vi "EOG_cancel_Method.vi"() -> ()   [LabVIEW 2014]
uses:
  <vilib>/Analysis/3filter.llb/Filter Passband Type.ctl
  <vilib>/Analysis/baseanly.llb/Real A x B.vi
  <vilib>/Utility/file.llb/Read From Spreadsheet File (DBL).vi
  <vilib>/Utility/file.llb/Read From Spreadsheet File (I64).vi
  <vilib>/Analysis/3filter.llb/Butterworth Filter (DBL).vi
  <vilib>/Analysis/Matrix/Numeric/Absolute Value/Absolute Value - RM.vi
  <vilib>/Analysis/Matrix/Numeric/Conversions/Matrix To Array - RM.vi
  <vilib>/Analysis/NI_AALBase.lvlib
  <vilib>/gmath/NI_Gmath.lvlib
  <vilib>/Analysis/Matrix/NI_Matrix.lvlib
panel:
  out "Revised 2":dbl[][](graph)
  in  "Cluster":path
  out "Revised":dbl[](graph)
  in  "Inverse_W":path
  out "Trans\nSTFT":dbl[][](graph)
  out "STFT":dbl[][](graph)
  in  "Exit":bool
  in  "Continuous/Discreet":bool
  in  "Forward":bool
  in  "Pause":bool
  out "STD Method":bool
  out "Cancel out \n(Std method)":dbl[](graph)
  out "Original":bool
  out "EEG":dbl[](graph)
  in  "Process":bool
  out "Processing":bool
  in  "Trial Number":i32=1
  in  "?":bool
  in  "Frame_Length":i32=20
  in  "Flash_Repeat":i32=20
  in  "Random_num":i32=6
  in  "EEG Data":path
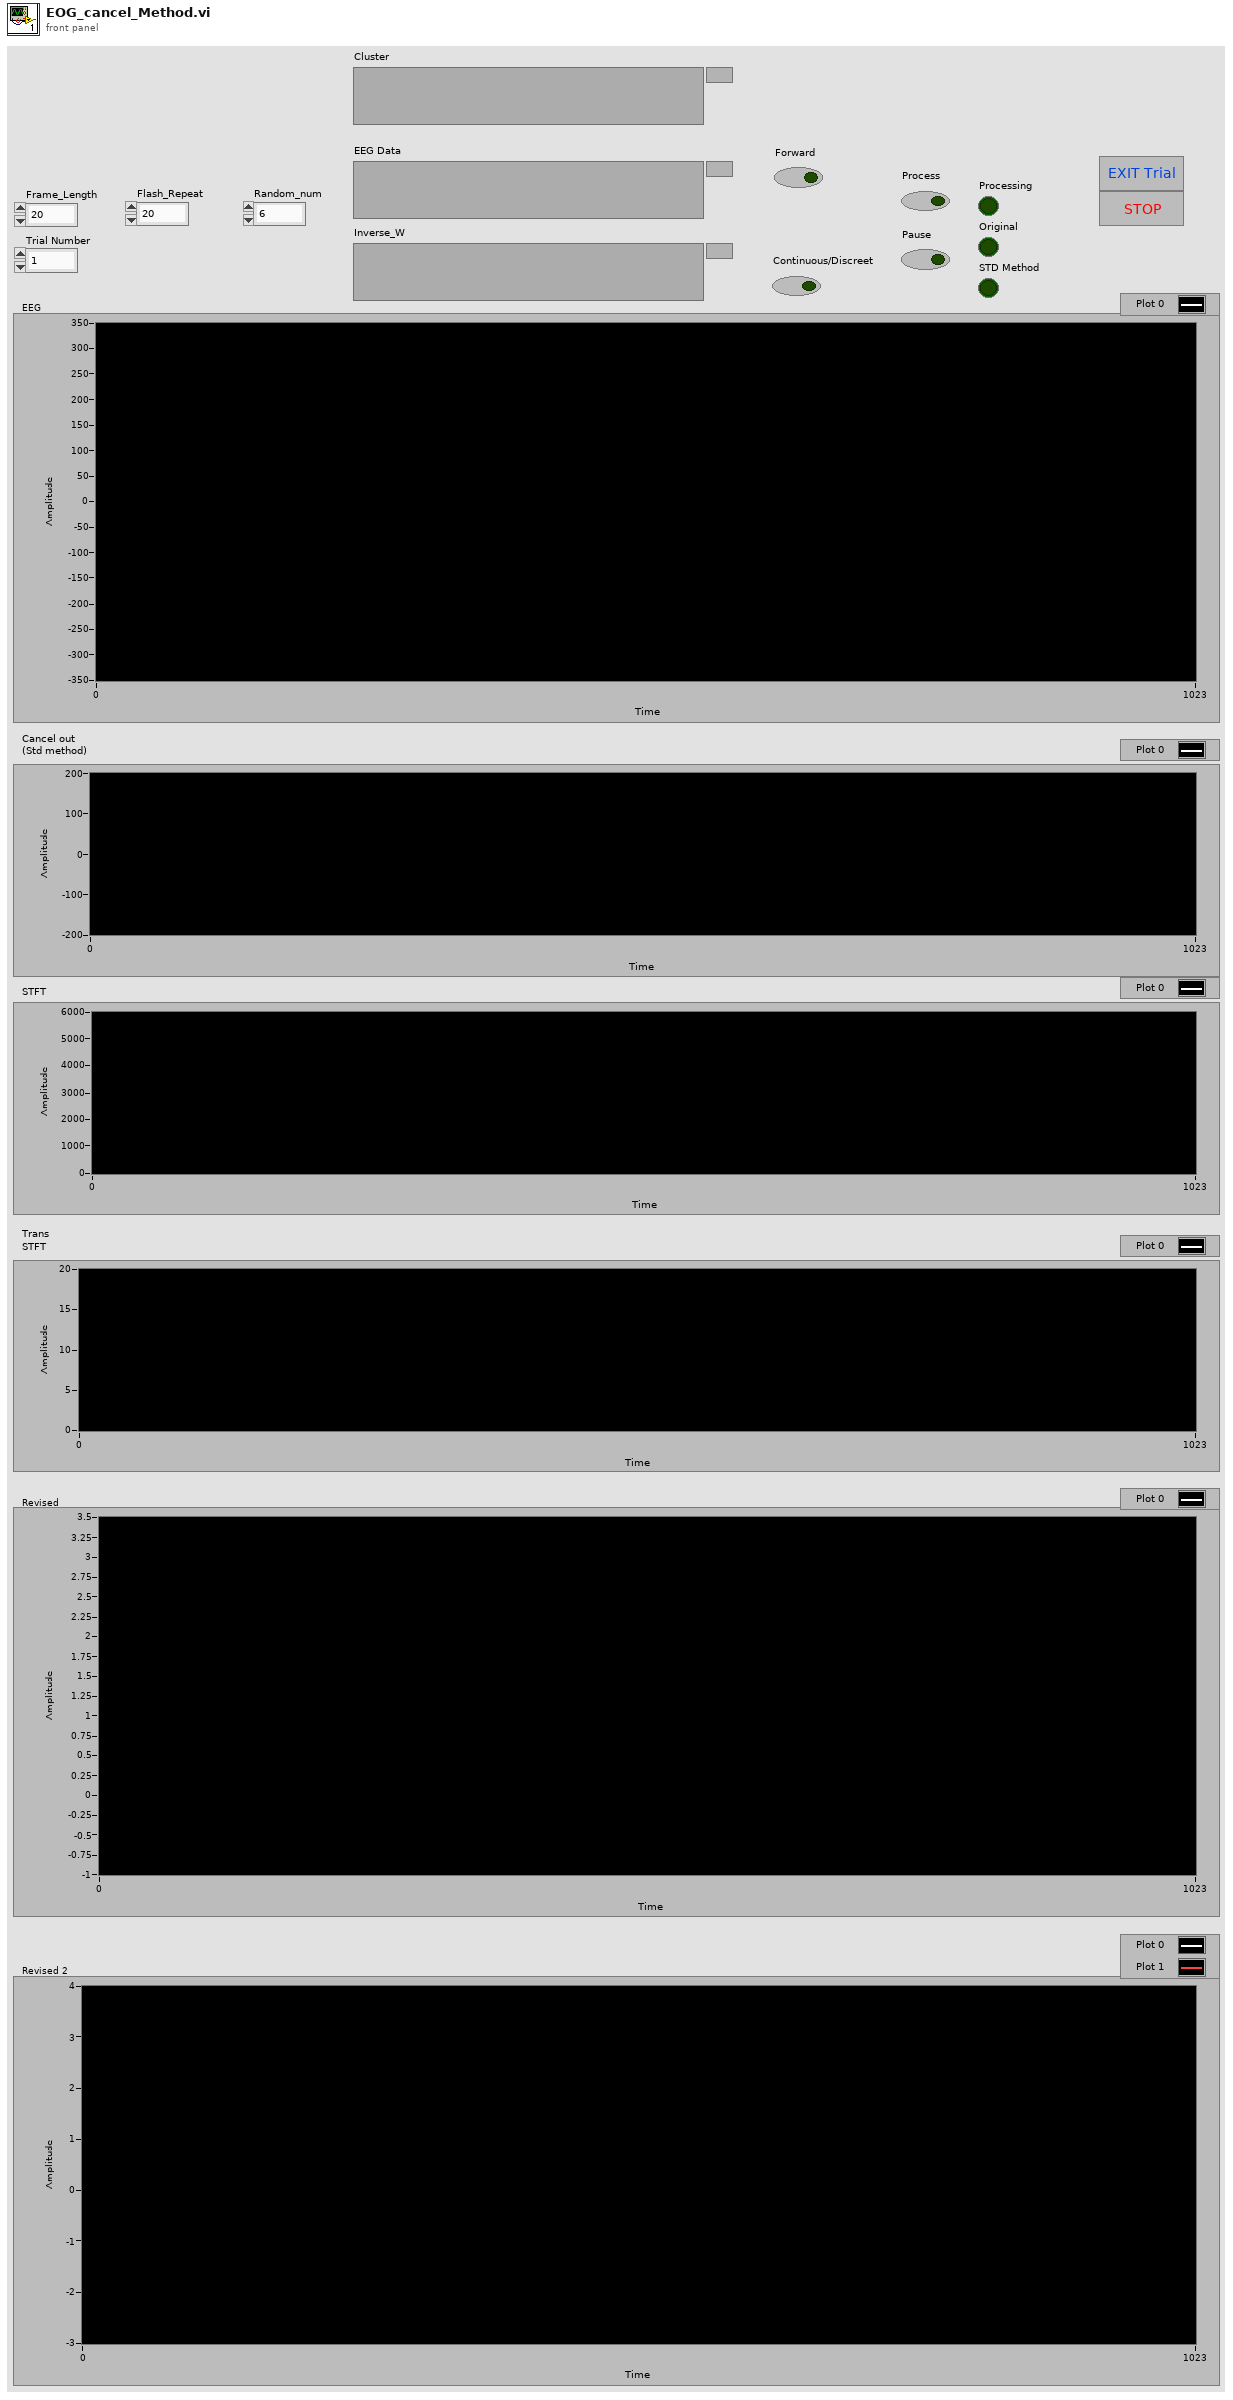
[diagram p1: front panel]
types:
  T1 = typedef "NI_AALBase.lvlib/Filter Passband Type.ctl" = enum32{"Lowpass", "Highpass", "Bandpass", "Bandstop"}
  T2 = typedef "NI_Matrix.lvlib/RealMatrix.ctl" = dbl[][]
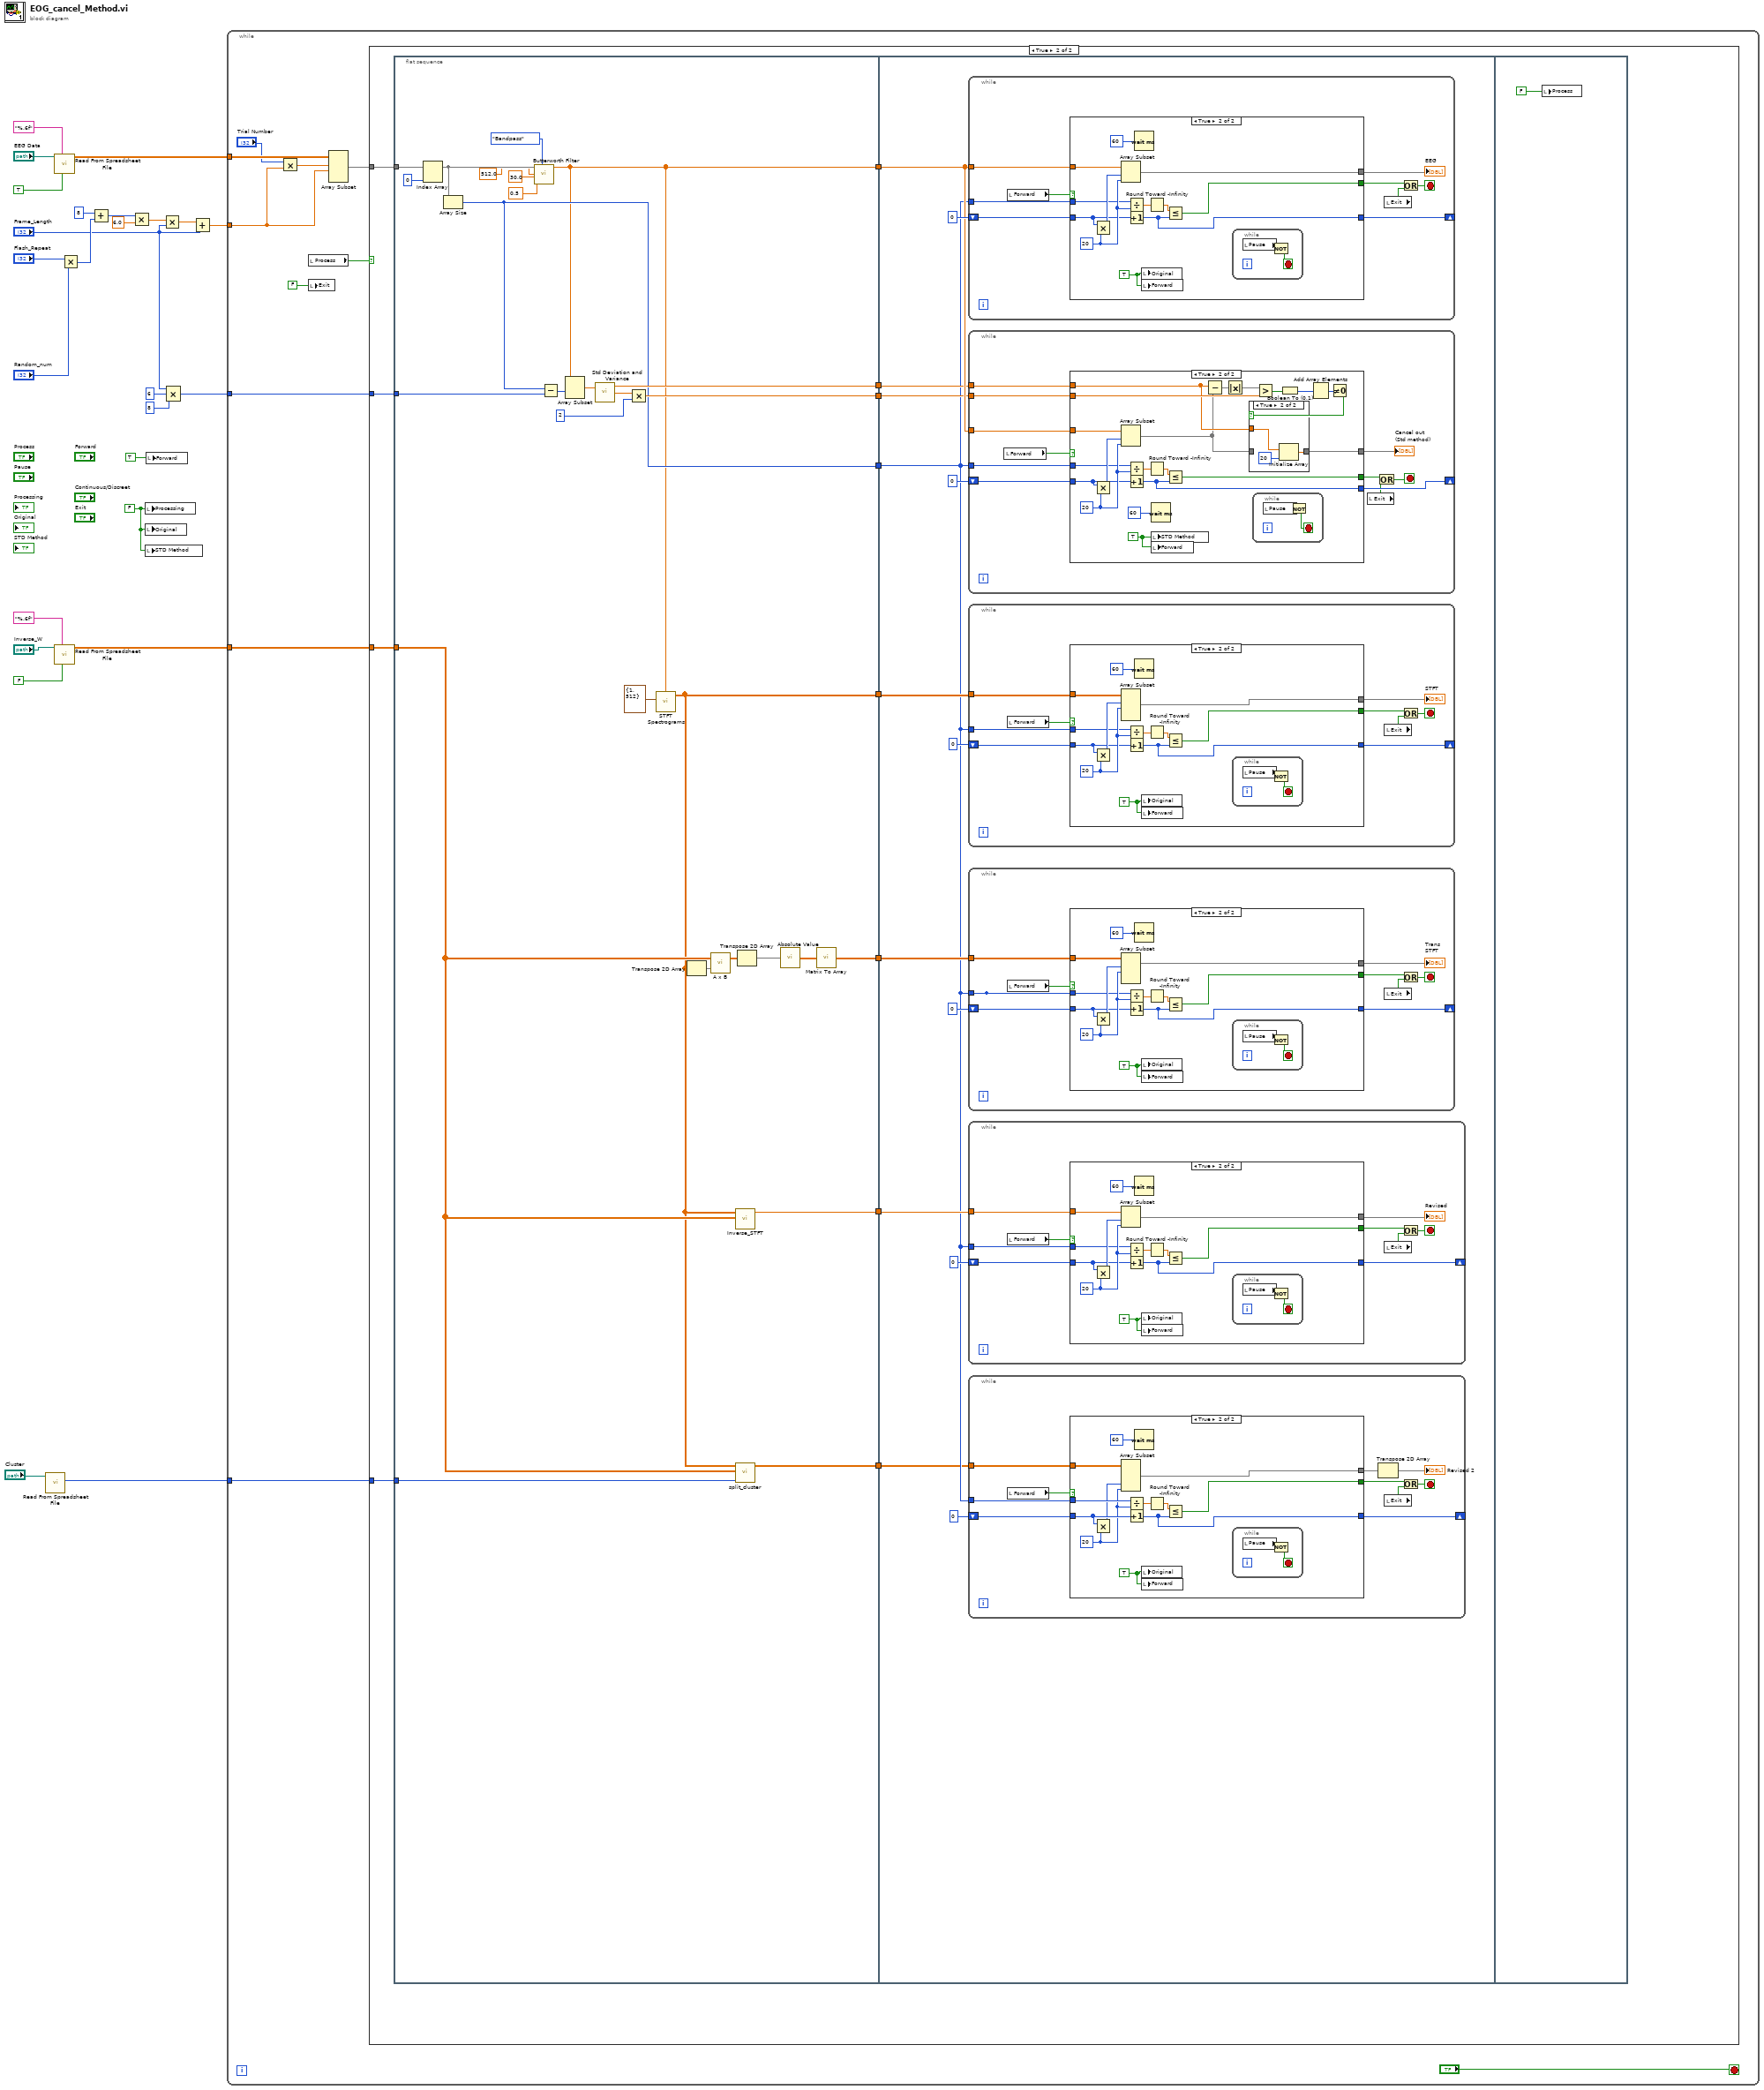
[diagram p0: block diagram]
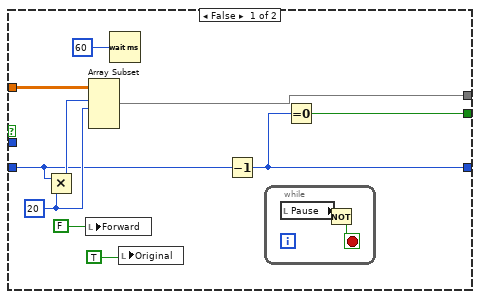
[diagram p3: hidden frame]
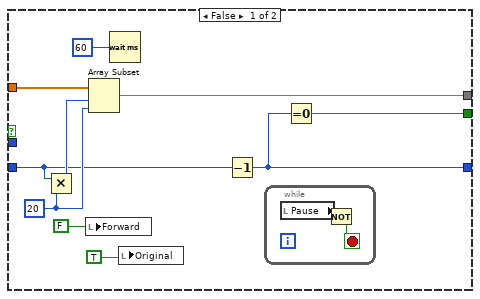
[diagram p4: hidden frame]
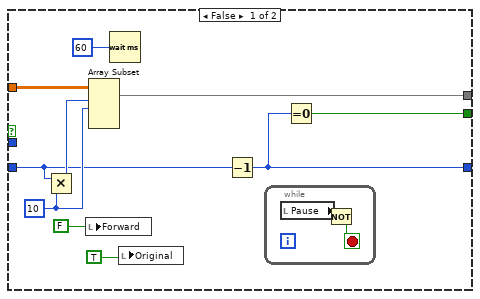
[diagram p5: hidden frame]
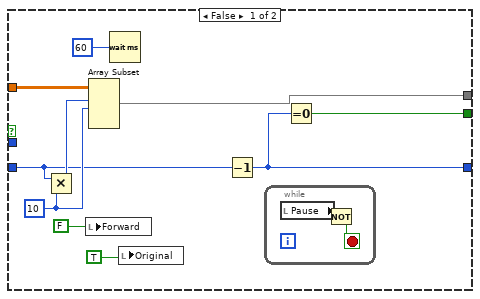
[diagram p6: hidden frame]
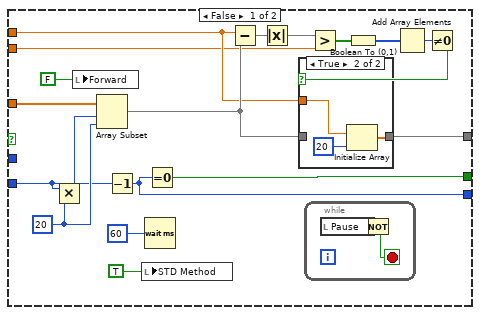
[diagram p7: hidden frame]
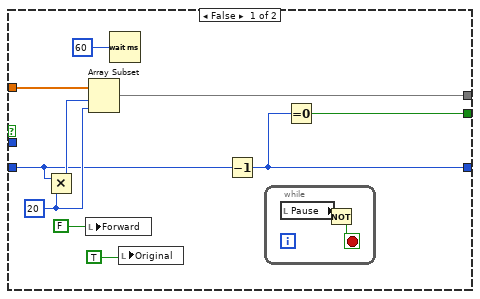
[diagram p10: hidden frame]
diagram:
  w7 = FALSE ("Processing")
  n1 = call-poly <vilib>:"Read From Spreadsheet File.vi"("file path (dialog if empty)"="Cluster") -> ("first row"=w1:i64[])  [unwired: 6 in, 4 out]
  n2 = call-poly <vilib>:"Read From Spreadsheet File.vi"("transpose (no:F)"=TRUE, "format (%.3f)"="%.6f", "file path (dialog if empty)"="EEG Data") -> ("all rows"=w13:dbl[][])  [unwired: 4 in, 4 out]
  n3 = call-poly <vilib>:"Read From Spreadsheet File.vi"("transpose (no:F)"=FALSE, "format (%.3f)"="%.6f", "file path (dialog if empty)"="Inverse_W") -> ("all rows"=w3:dbl[][])  [unwired: 4 in, 4 out]
  n4 = Multiply(x="Flash_Repeat", y="Random_num") -> (x*y=w17:i32)
  n5 = Add(x=8, y=w17) -> (x+y=w19:i32)
  n6 = Multiply(x=w19, y=6.0) -> (x*y=w21:dbl)
  n7 = local write "Processing"(w7) -> ()
  n8 = local write "Original"(w7) -> ()
  n9 = local write "STD Method"(w7) -> ()
  n10 = local write "Forward"(TRUE ("Forward")) -> ()
  n11 = Multiply(x=w21, y="Frame_Length") -> (x*y=w22:dbl)
  n12 = Compound Arithmetic op=MULTIPLY("Frame_Length", 6 ("x"), 8 ("x")) -> (w9:i32)
  n13 = Add(x=w22, y="Frame_Length") -> (x+y=w14:dbl)
  n14 = while {
    tunnel: w13 -> [w35]
    tunnel: w14 -> [w33]
    tunnel: w9 -> [w30]
    tunnel: w3 -> [w27]
    tunnel: w1 -> [w26]
    stop <- "?" stop-if-true
    n15 = Multiply(x="Trial Number", y=w33) -> (x*y=w34:dbl)
    n16 = local read "Process"() -> (w29:bool)
    n17 = local write "Exit"(FALSE ("Exit")) -> ()
    n18 = Array Subset(array=w35, index (row)=w34, length (row)=w33) -> (w31:dbl[][])  [unwired: 2 in]
    n19 = case shown="True" w29 {
      tunnel: w31 -> [_ w47]
      tunnel: w30 -> [_ w48]
      tunnel: w27 -> [_ w46]
      tunnel: w26 -> [_ w38]
      frame False {
      }
      frame True {
        n20 = flat-sequence {
          tunnel: w48 -> [w75]
          tunnel: w47 -> [w74]
          tunnel: w46 -> [w50]
          tunnel: [w70] -> w45
          tunnel: [w69] -> w44
          tunnel: [w61] -> w43
          tunnel: [w59] -> w42
          tunnel: [w49] -> w41
          tunnel: [w53] -> w40
          tunnel: [w55] -> w39
          tunnel: w38 -> [w52]
          tunnel: [w51] -> w37
          tunnel: w45 -> [w84]
          tunnel: w44 -> [w85]
          tunnel: w43 -> [w77]
          tunnel: w42 -> [w86]
          tunnel: w41 -> [w83]
          tunnel: w40 -> [w82]
          tunnel: w39 -> [w79]
          tunnel: w37 -> [w76]
          frame #0 {
            n21 = Index Array(array=w74, index (col)=0 ("disabled index (col)")) -> (element=w64:dbl[])  [unwired: 1 in]
            n22 = Array Size(array=w64) -> (size(s)=w61:i32)
            n23 = call-poly <vilib>:"Butterworth Filter.vi"("filter type"=Filter_Passband_Type."Bandpass", "low cutoff freq: fl"=0.5, "high cutoff freq: fh"=30.0, "sampling freq: fs"=512.0 ("high cutoff freq: fh"), "X"=w64) -> ("Filtered X"=w59:dbl[])  [unwired: 3 in, 1 out]
            n24 = Subtract(x=w61, y=w75) -> (x-y=w73:i32)
            n25 = Array Subset(array=w59, index=w73) -> (w62:dbl[])  [unwired: 1 in]
            n26 = call <vilib>:"Std Deviation and Variance.vi"("X"=w62) -> ("mean"=w69:dbl, "standard deviation"=w72:dbl)  [unwired: 1 in, 1 out]
            n27 = Multiply(x=w72, y=2 ("disabled index (col)")) -> (x*y=w70:dbl)
            n28 = call <vilib>:"STFT Spectrograms.vi"("time-freq sampling info"=cluster{"time steps":i32, "frequency bins":i32} {"time steps"=1, "frequency bins"=512}, "X"=w59) -> ("STFT Spectrogram {X}"=w49:dbl[][])  [unwired: 8 in, 1 out]
            n29 = Transpose 2D Array(2D array=w49) -> (transposed array=w58:dbl[][])
            n30 = call-poly <vilib>:"A x B.vi"("B"=w58, "A"=w50) -> ("A x B"=w56:T2)  [unwired: 1 out]
            n31 = call "Inverse_STFT.vi"("W"=w50, "STFT Spectrogram {X}"=w49) -> ("Inverse_STFT"=w55:dbl[])  [unwired: 9 in]
            n32 = call "split_cluster.vi"("Clustering"=w52, "W"=w50, "STFT Spectrogram {X}"=w49) -> ("Splited_X(t)"=w51:dbl[][])  [unwired: 7 in, 1 out]
            n33 = Transpose 2D Array(2D array=w56) -> (transposed array=w57:T2)
            n34 = call-poly <vilib>:"Absolute Value.vi"("Real Matrix A"=w57) -> ("|A|"=w54:T2)
            n35 = call-poly <vilib>:"Matrix To Array.vi"("Real Matrix"=w54) -> ("Real 2D Array"=w53:dbl[][])
          }
          frame #1 {
            n36 = while {
              tunnel: w86 -> [w302]
              tunnel: w77 -> [w301]
              shift-right: [w299] -> _
              shift-left: 0 ("disabled index (col)") -> [w300]
              stop <- w297 stop-if-true
              n37 = local read "Forward"() -> (w294:bool)
              n38 = case shown="True" w294 {
                tunnel: w302 -> [w309 w326]
                tunnel: w301 -> [_ w321]
                tunnel: [w306 w320] -> w296
                tunnel: w300 -> [w307 w318]
                tunnel: [w305 w316] -> w299
                tunnel: [w308 w317] -> w298
                frame False {
                  w311 = 20
                  n39 = Multiply(x=w307, y=w311) -> (x*y=w312:i32)
                  n40 = local write "Forward"(FALSE ("Forward")) -> ()
                  n41 = Array Subset(array=w309, index=w312, length=w311) -> (w308:dbl[])
                  n42 = Wait (ms)(milliseconds to wait=u32 60) -> ()  [unwired: 1 out]
                  n43 = local write "Original"(TRUE ("Processing")) -> ()
                  n44 = Decrement(x=w307) -> (x-1=w305:i32)
                  n45 = while {
                    stop <- w313 stop-if-true
                    n46 = local read "Pause"() -> (w314:bool)
                    n47 = Not(x=w314) -> (.not. x?=w313:bool)
                  }
                  n48 = Equal To 0?(x=w305) -> (x = 0?=w306:bool)
                }
                frame True {
                  w315 = TRUE ("Processing")
                  w322 = 20
                  n49 = Multiply(x=w318, y=w322) -> (x*y=w325:i32)
                  n50 = Array Subset(array=w326, index=w325, length=w322) -> (w317:dbl[])
                  n51 = Divide(x=w321, y=w322) -> (x/y=w323:dbl)
                  n52 = Increment(x=w318) -> (x+1=w316:i32)
                  n53 = Wait (ms)(milliseconds to wait=u32 60) -> ()  [unwired: 1 out]
                  n54 = local write "Original"(w315) -> ()
                  n55 = local write "Forward"(w315) -> ()
                  n56 = Round Toward -Infinity(1:w323) -> (0:w324:dbl)
                  n57 = Less Or Equal?(x=w324, y=w316) -> (x <= y?=w320:bool)
                  n58 = while {
                    stop <- w327 stop-if-true
                    n59 = local read "Pause"() -> (w328:bool)
                    n60 = Not(x=w328) -> (.not. x?=w327:bool)
                  }
                }
              }
              "EEG" <- w298
              n61 = local read "Exit"() -> (w295:bool)
              n62 = Or(x=w296, y=w295) -> (x .or. y?=w297:bool)
            }
            n63 = while {
              tunnel: w86 -> [w241]
              tunnel: w77 -> [w240]
              tunnel: w84 -> [w238]
              tunnel: w85 -> [w237]
              shift-right: [w235] -> _
              shift-left: 0 ("disabled index (col)") -> [w236]
              stop <- w233 stop-if-true
              n64 = local read "Forward"() -> (w231:bool)
              n65 = case shown="True" w231 {
                tunnel: w241 -> [w248 w287]
                tunnel: w240 -> [_ w282]
                tunnel: [w244 w281] -> w234
                tunnel: [w247 w279] -> w239
                tunnel: w238 -> [w250 w276]
                tunnel: w237 -> [w251 w271]
                tunnel: w236 -> [w246 w269]
                tunnel: [w245 w268] -> w235
                frame False {
                  w259 = 20
                  n66 = Multiply(x=w246, y=w259) -> (x*y=w260:i32)
                  n67 = local write "Forward"(FALSE ("Forward")) -> ()
                  n68 = Array Subset(array=w248, index=w260, length=w259) -> (w252:dbl[])
                  n69 = Decrement(x=w246) -> (x-1=w245:i32)
                  n70 = local write "STD Method"(TRUE ("Processing")) -> ()
                  n71 = Wait (ms)(milliseconds to wait=u32 60) -> ()  [unwired: 1 out]
                  n72 = Equal To 0?(x=w245) -> (x = 0?=w244:bool)
                  n73 = Subtract(x=w252, y=w251) -> (x-y=w257:dbl[])
                  n74 = Absolute Value(x=w257) -> (abs(x)=w256:dbl[])
                  n75 = while {
                    stop <- w261 stop-if-true
                    n76 = local read "Pause"() -> (w262:bool)
                    n77 = Not(x=w262) -> (.not. x?=w261:bool)
                  }
                  n78 = Greater?(x=w256, y=w250) -> (0:w255:bool[])
                  n79 = Boolean To (0,1)(Boolean=w255) -> (0, 1=w249:i16[])
                  n80 = Add Array Elements(numeric array=w249) -> (sum=w254:i16)
                  n81 = Not Equal To 0?(x=w254) -> (x != 0?=w253:bool)
                  n82 = case shown="True" w253 {
                    tunnel: w252 -> [w263 _]
                    tunnel: [w263 w266] -> w247
                    tunnel: w251 -> [_ w264]
                    frame False {
                    }
                    frame True {
                      n83 = Initialize Array(w264, 20 ("dimension size")) -> (w266:dbl[])
                    }
                  }
                }
                frame True {
                  w267 = TRUE ("Processing")
                  w283 = 20
                  n84 = Multiply(x=w269, y=w283) -> (x*y=w286:i32)
                  n85 = Array Subset(array=w287, index=w286, length=w283) -> (w270:dbl[])
                  n86 = Divide(x=w282, y=w283) -> (x/y=w284:dbl)
                  n87 = Increment(x=w269) -> (x+1=w268:i32)
                  n88 = Round Toward -Infinity(1:w284) -> (0:w285:dbl)
                  n89 = Wait (ms)(milliseconds to wait=u32 60) -> ()  [unwired: 1 out]
                  n90 = local write "STD Method"(w267) -> ()
                  n91 = local write "Forward"(w267) -> ()
                  n92 = Less Or Equal?(x=w285, y=w268) -> (x <= y?=w281:bool)
                  n93 = Subtract(x=w270, y=w271) -> (x-y=w278:dbl[])
                  n94 = Absolute Value(x=w278) -> (abs(x)=w277:dbl[])
                  n95 = while {
                    stop <- w288 stop-if-true
                    n96 = local read "Pause"() -> (w289:bool)
                    n97 = Not(x=w289) -> (.not. x?=w288:bool)
                  }
                  n98 = Greater?(x=w277, y=w276) -> (0:w275:bool[])
                  n99 = Boolean To (0,1)(Boolean=w275) -> (0, 1=w274:i16[])
                  n100 = Add Array Elements(numeric array=w274) -> (sum=w273:i16)
                  n101 = Not Equal To 0?(x=w273) -> (x != 0?=w272:bool)
                  n102 = case shown="True" w272 {
                    tunnel: w270 -> [w290 _]
                    tunnel: [w290 w293] -> w279
                    tunnel: w271 -> [_ w291]
                    frame False {
                    }
                    frame True {
                      n103 = Initialize Array(w291, 20 ("dimension size")) -> (w293:dbl[])
                    }
                  }
                }
              }
              "Cancel out \n(Std method)" <- w239
              n104 = local read "Exit"() -> (w232:bool)
              n105 = Or(x=w234, y=w232) -> (x .or. y?=w233:bool)
            }
            n106 = while {
              tunnel: w83 -> [w204]
              tunnel: w77 -> [w203]
              shift-right: [w201] -> _
              shift-left: 0 ("disabled index (col)") -> [w202]
              stop <- w199 stop-if-true
              n107 = local read "Forward"() -> (w196:bool)
              n108 = case shown="True" w196 {
                tunnel: w204 -> [w211 w228]
                tunnel: w203 -> [_ w223]
                tunnel: [w208 w222] -> w198
                tunnel: w202 -> [w209 w220]
                tunnel: [w207 w218] -> w201
                tunnel: [w210 w219] -> w200
                frame False {
                  w213 = 10
                  n109 = Multiply(x=w209, y=w213) -> (x*y=w214:i32)
                  n110 = local write "Forward"(FALSE ("Forward")) -> ()
                  n111 = Array Subset(array=w211, index (row)=w214, length (row)=w213) -> (w210:dbl[][])  [unwired: 2 in]
                  n112 = Wait (ms)(milliseconds to wait=u32 60) -> ()  [unwired: 1 out]
                  n113 = local write "Original"(TRUE ("Processing")) -> ()
                  n114 = Decrement(x=w209) -> (x-1=w207:i32)
                  n115 = while {
                    stop <- w215 stop-if-true
                    n116 = local read "Pause"() -> (w216:bool)
                    n117 = Not(x=w216) -> (.not. x?=w215:bool)
                  }
                  n118 = Equal To 0?(x=w207) -> (x = 0?=w208:bool)
                }
                frame True {
                  w217 = TRUE ("Processing")
                  w224 = 20
                  n119 = Multiply(x=w220, y=w224) -> (x*y=w227:i32)
                  n120 = Array Subset(array=w228, index (row)=w227, length (row)=w224) -> (w219:dbl[][])  [unwired: 2 in]
                  n121 = Divide(x=w223, y=w224) -> (x/y=w225:dbl)
                  n122 = Increment(x=w220) -> (x+1=w218:i32)
                  n123 = Wait (ms)(milliseconds to wait=u32 60) -> ()  [unwired: 1 out]
                  n124 = local write "Original"(w217) -> ()
                  n125 = local write "Forward"(w217) -> ()
                  n126 = Round Toward -Infinity(1:w225) -> (0:w226:dbl)
                  n127 = Less Or Equal?(x=w226, y=w218) -> (x <= y?=w222:bool)
                  n128 = while {
                    stop <- w229 stop-if-true
                    n129 = local read "Pause"() -> (w230:bool)
                    n130 = Not(x=w230) -> (.not. x?=w229:bool)
                  }
                }
              }
              "STFT" <- w200
              n131 = local read "Exit"() -> (w197:bool)
              n132 = Or(x=w198, y=w197) -> (x .or. y?=w199:bool)
            }
            n133 = while {
              tunnel: w82 -> [w169]
              tunnel: w77 -> [w161]
              shift-right: [w167] -> _
              shift-left: 0 ("disabled index (col)") -> [w168]
              tunnel: [w161] -> _
              stop <- w165 stop-if-true
              n134 = local read "Forward"() -> (w162:bool)
              n135 = case shown="True" w162 {
                tunnel: w169 -> [w176 w193]
                tunnel: w161 -> [_ w188]
                tunnel: [w173 w187] -> w164
                tunnel: w168 -> [w174 w185]
                tunnel: [w172 w184] -> w167
                tunnel: [w175 w182] -> w166
                frame False {
                  w178 = 10
                  n136 = Multiply(x=w174, y=w178) -> (x*y=w179:i32)
                  n137 = local write "Forward"(FALSE ("Forward")) -> ()
                  n138 = Array Subset(array=w176, index (row)=w179, length (row)=w178) -> (w175:dbl[][])  [unwired: 2 in]
                  n139 = Wait (ms)(milliseconds to wait=u32 60) -> ()  [unwired: 1 out]
                  n140 = local write "Original"(TRUE ("Processing")) -> ()
                  n141 = Decrement(x=w174) -> (x-1=w172:i32)
                  n142 = while {
                    stop <- w180 stop-if-true
                    n143 = local read "Pause"() -> (w181:bool)
                    n144 = Not(x=w181) -> (.not. x?=w180:bool)
                  }
                  n145 = Equal To 0?(x=w172) -> (x = 0?=w173:bool)
                }
                frame True {
                  w183 = TRUE ("Processing")
                  w189 = 20
                  n146 = Multiply(x=w185, y=w189) -> (x*y=w192:i32)
                  n147 = Array Subset(array=w193, index (row)=w192, length (row)=w189) -> (w182:dbl[][])  [unwired: 2 in]
                  n148 = Divide(x=w188, y=w189) -> (x/y=w190:dbl)
                  n149 = Increment(x=w185) -> (x+1=w184:i32)
                  n150 = Wait (ms)(milliseconds to wait=u32 60) -> ()  [unwired: 1 out]
                  n151 = local write "Original"(w183) -> ()
                  n152 = local write "Forward"(w183) -> ()
                  n153 = Round Toward -Infinity(1:w190) -> (0:w191:dbl)
                  n154 = Less Or Equal?(x=w191, y=w184) -> (x <= y?=w187:bool)
                  n155 = while {
                    stop <- w194 stop-if-true
                    n156 = local read "Pause"() -> (w195:bool)
                    n157 = Not(x=w195) -> (.not. x?=w194:bool)
                  }
                }
              }
              "Trans\nSTFT" <- w166
              n158 = local read "Exit"() -> (w163:bool)
              n159 = Or(x=w164, y=w163) -> (x .or. y?=w165:bool)
            }
            n160 = while {
              tunnel: w79 -> [w134]
              tunnel: w77 -> [w133]
              shift-right: [w131] -> _
              shift-left: 0 ("disabled index (col)") -> [w132]
              stop <- w129 stop-if-true
              n161 = local read "Forward"() -> (w126:bool)
              n162 = case shown="True" w126 {
                tunnel: w134 -> [w141 w158]
                tunnel: w133 -> [_ w153]
                tunnel: [w138 w152] -> w128
                tunnel: w132 -> [w139 w150]
                tunnel: [w137 w148] -> w131
                tunnel: [w140 w149] -> w130
                frame False {
                  w143 = 20
                  n163 = Multiply(x=w139, y=w143) -> (x*y=w144:i32)
                  n164 = local write "Forward"(FALSE ("Forward")) -> ()
                  n165 = Array Subset(array=w141, index=w144, length=w143) -> (w140:dbl[])
                  n166 = Wait (ms)(milliseconds to wait=u32 60) -> ()  [unwired: 1 out]
                  n167 = local write "Original"(TRUE ("Processing")) -> ()
                  n168 = Decrement(x=w139) -> (x-1=w137:i32)
                  n169 = while {
                    stop <- w145 stop-if-true
                    n170 = local read "Pause"() -> (w146:bool)
                    n171 = Not(x=w146) -> (.not. x?=w145:bool)
                  }
                  n172 = Equal To 0?(x=w137) -> (x = 0?=w138:bool)
                }
                frame True {
                  w147 = TRUE ("Processing")
                  w154 = 20
                  n173 = Multiply(x=w150, y=w154) -> (x*y=w157:i32)
                  n174 = Array Subset(array=w158, index=w157, length=w154) -> (w149:dbl[])
                  n175 = Divide(x=w153, y=w154) -> (x/y=w155:dbl)
                  n176 = Increment(x=w150) -> (x+1=w148:i32)
                  n177 = Wait (ms)(milliseconds to wait=u32 60) -> ()  [unwired: 1 out]
                  n178 = local write "Original"(w147) -> ()
                  n179 = local write "Forward"(w147) -> ()
                  n180 = Round Toward -Infinity(1:w155) -> (0:w156:dbl)
                  n181 = Less Or Equal?(x=w156, y=w148) -> (x <= y?=w152:bool)
                  n182 = while {
                    stop <- w159 stop-if-true
                    n183 = local read "Pause"() -> (w160:bool)
                    n184 = Not(x=w160) -> (.not. x?=w159:bool)
                  }
                }
              }
              "Revised" <- w130
              n185 = local read "Exit"() -> (w127:bool)
              n186 = Or(x=w128, y=w127) -> (x .or. y?=w129:bool)
            }
            n187 = while {
              tunnel: w76 -> [w99]
              tunnel: w77 -> [w98]
              shift-right: [w96] -> _
              shift-left: 0 -> [w97]
              stop <- w95 stop-if-true
              n188 = local read "Forward"() -> (w92:bool)
              n189 = case shown="True" w92 {
                tunnel: w99 -> [w106 w123]
                tunnel: w98 -> [_ w120]
                tunnel: [w103 w119] -> w94
                tunnel: w97 -> [w104 w117]
                tunnel: [w102 w115] -> w96
                tunnel: [w105 w116] -> w91
                frame False {
                  w108 = 20
                  n190 = Multiply(x=w104, y=w108) -> (x*y=w109:i32)
                  n191 = local write "Forward"(FALSE ("Forward")) -> ()
                  n192 = Array Subset(array=w106, index (row)=w109, length (row)=w108) -> (w105:dbl[][])  [unwired: 2 in]
                  n193 = Wait (ms)(milliseconds to wait=u32 60) -> ()  [unwired: 1 out]
                  n194 = local write "Original"(TRUE ("Processing")) -> ()
                  n195 = Decrement(x=w104) -> (x-1=w102:i32)
                  n196 = while {
                    stop <- w110 stop-if-true
                    n197 = local read "Pause"() -> (w111:bool)
                    n198 = Not(x=w111) -> (.not. x?=w110:bool)
                  }
                  n199 = Equal To 0?(x=w102) -> (x = 0?=w103:bool)
                }
                frame True {
                  w114 = TRUE ("Processing")
                  w112 = 20
                  n200 = Multiply(x=w117, y=w112) -> (x*y=w113:i32)
                  n201 = Array Subset(array=w123, index (col)=w113, length (col)=w112) -> (w116:dbl[][])  [unwired: 2 in]
                  n202 = Divide(x=w120, y=w112) -> (x/y=w121:dbl)
                  n203 = Increment(x=w117) -> (x+1=w115:i32)
                  n204 = Wait (ms)(milliseconds to wait=u32 60) -> ()  [unwired: 1 out]
                  n205 = local write "Original"(w114) -> ()
                  n206 = local write "Forward"(w114) -> ()
                  n207 = Round Toward -Infinity(1:w121) -> (0:w122:dbl)
                  n208 = Less Or Equal?(x=w122, y=w115) -> (x <= y?=w119:bool)
                  n209 = while {
                    stop <- w124 stop-if-true
                    n210 = local read "Pause"() -> (w125:bool)
                    n211 = Not(x=w125) -> (.not. x?=w124:bool)
                  }
                }
              }
              n212 = Transpose 2D Array(2D array=w91) -> (transposed array=→"Revised 2":dbl[][])
              n213 = local read "Exit"() -> (w93:bool)
              n214 = Or(x=w94, y=w93) -> (x .or. y?=w95:bool)
            }
          }
          frame #2 {
            n215 = local write "Process"(FALSE ("Processing")) -> ()
          }
        }
      }
    }
  }
